vi "note.vi"(10 "user event":refnum<user-event>) -> ()   [LabVIEW 2017]
panel:
  # "Processing SVN command\nPlease wait - that will take a while..."
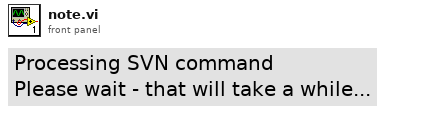
[diagram p1: front panel]
types:
  T1 = enum32{"Invalid", "Standard", "Closed", "Hidden", "Minimized", "Maximized"}
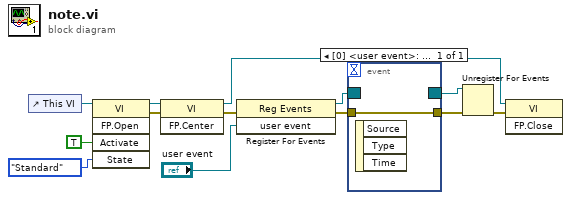
[diagram p0: block diagram]
diagram:
  n1 = control-ref of="This VI"() -> (w12:refnum<vi>)
  n2 = invoke class="VI" method="FP.Open"(reference=w12, "Activate"=TRUE ("Activate?"), "State"=T1."Standard") -> (reference out=w9:refnum<vi>, error out=w8:errorcluster)  [unwired: 2 in, 3 out]
  n3 = invoke class="VI" method="FP.Center"(reference=w9, error in=w8) -> (reference out=w2:refnum<vi>, error out=w7:errorcluster)  [unwired: 1 in, 1 out]
  n4 = register-events(error in=w7, "user event") -> (reference out=w13:refnum<event-registration>, error out=w6:errorcluster)  [unwired: 1 in]
  n5 = event shown="[0] <user event>: User Event" {
    selector: w13 -> [_]
    dyn-events: [_] -> w5
    timeout: _ -> [_]
    tunnel: w6 -> [w14]
    tunnel: [w14] -> w4
    event User Event {
      n6 = event-data() -> ()  [unwired: 1 in, 3 out]
    }
  }
  n7 = Unregister For Events(event registration refnum=w5, error in=w4) -> (error out=w3:errorcluster)
  n8 = invoke class="VI" method="FP.Close"(reference=w2, error in=w3) -> ()  [unwired: 1 in, 3 out]
